vi "compare Image In Cyclone With File.vi"(8 "error in":errorcluster, 9 "imageId":u32, 10 "aFile":string, 11 "cycloneHandle":u32) -> (0 "error out":errorcluster, 2 "aFile out":string, 3 "function return":bool)   [LabVIEW 2021, in "CycloneControlSDK.lvlib"]
doc: "extern \"C\" bool _cdecl compareImageInCycloneWithFile(uint32_t cycloneHandle, char *aFile, uint32_t imageId);"
uses:
  CycloneControlSDK.lvlib
  CycloneControlSDK_64.dll
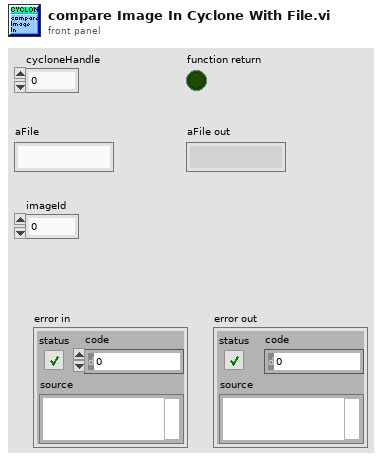
[diagram p1: front panel]
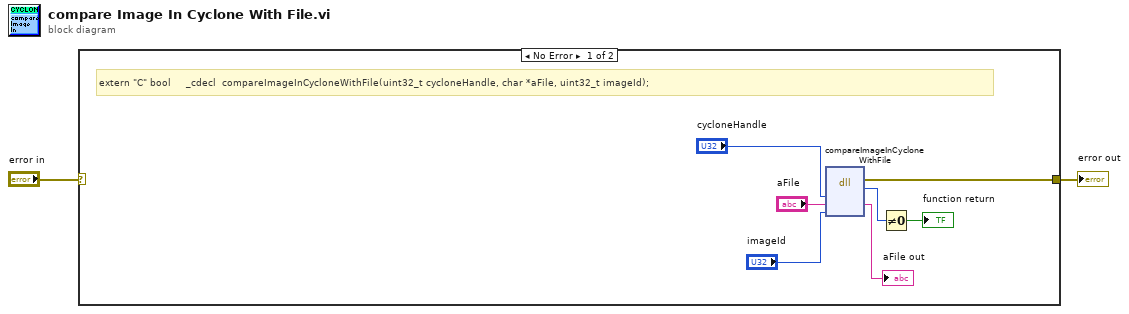
[diagram p0: block diagram]
diagram:
  n1 = case shown="No Error" "error in" {
    selector: "error in" -> [_ w10]
    tunnel: [w3 w10] -> w2
    frame No Error {
      # "extern \"C\" bool     _cdecl  compareImageInCycloneWithFile(uint32_t cycloneHandle, char *aFile, uint32_t imageId);"
      n2 = dll-call lib="C:/PEMicro/cyclone/cycloneControl/controlsdk/examples/labview2018/user.lib/CycloneControlSDK/CycloneControlSDK_64.dll" fn="compareImageInCycloneWithFile"("cycloneHandle"="cycloneHandle", "aFile"="aFile", "imageId"="imageId") -> (error out=w3:errorcluster, "return type"=w8:u8, "aFile"=→"aFile out":string)  [unwired: 5 in, 1 out]
      n3 = Not Equal To 0?(x=w8) -> (x != 0?=→"function return":bool)
    }
    frame Error {
    }
  }
  "error out" <- w2
